vi "func-gen-simple-motor-sim.vi"(9 "Current Position Ft":dbl, 11 "Motor-Demand":dbl) -> (1 "Updated Position Ft":dbl, 3 "Velocity Ft/Sec":dbl)   [LabVIEW 2019]
uses:
  <vilib>/Rock Robotics/WPI/ThirdParty/JAS_Junk/TrajLib/VI/Util_GetTime_U32.vi
  <vilib>/Rock Robotics/WPI/ThirdParty/JAS_Junk/TrajLib/VI/TimeInterpDouble_New.vi
  <vilib>/Rock Robotics/WPI/ThirdParty/JAS_Junk/TrajLib/VI/TimeInterpDouble_AddSample.vi
  <vilib>/Rock Robotics/WPI/ThirdParty/JAS_Junk/TrajLib/VI/TimeInterpDouble_GetSample.vi
  <vilib>/Rock Robotics/WPI/ThirdParty/JAS_Junk/TrajLib/VI/TimeInterpDouble_SetMaxTime.vi
  <vilib>/Rock Robotics/WPI/ThirdParty/JAS_Junk/TrajLib/VI/TimeInterpDouble_CleanUp.vi
  <vilib>/Rock Robotics/WPI/ThirdParty/JAS_Junk/TrajLib/MathUtil_Interpolate.vi
  <vilib>/Rock Robotics/WPI/ThirdParty/JAS_Junk/TrajLib/VI/Util_GetTime_U64.vi
  <vilib>/gmath/interp.llb/Search Ordered Table.vi
  <vilib>/Rock Robotics/WPI/ThirdParty/JAS_Junk/TrajLib/Trajectory_Library.lvlib
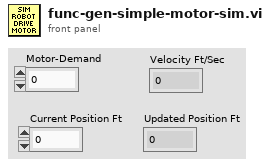
[diagram p1: front panel]
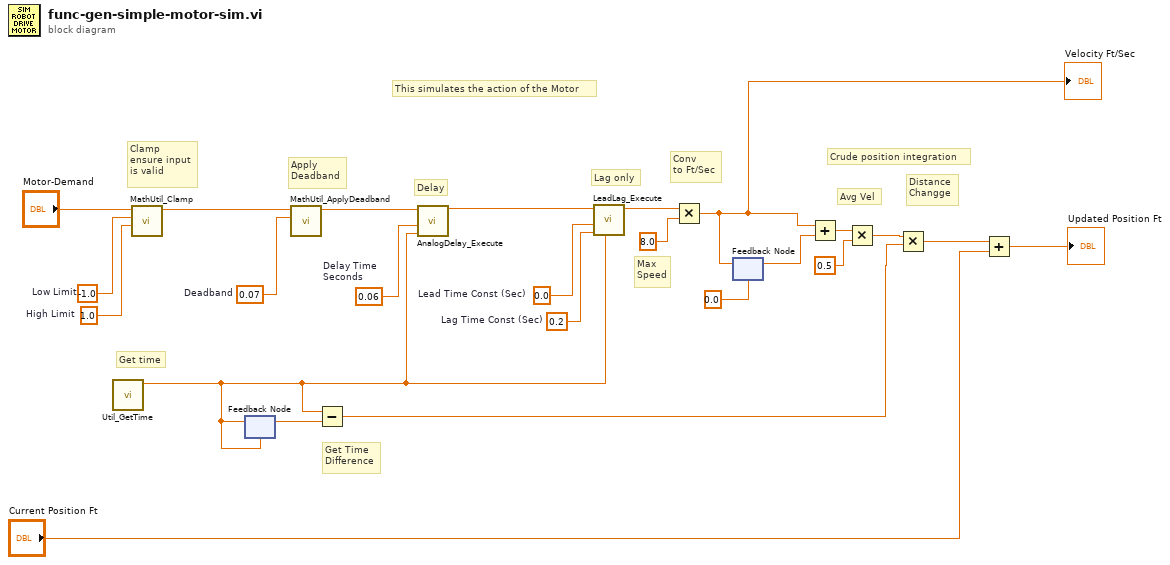
[diagram p0: block diagram]
diagram:
  w19 = 1.0  # High Limit
  w18 = -1.0  # Low Limit
  w21 = 0.2  # Lag Time Const (Sec)
  w20 = 0.0  # Lead Time Const (Sec)
  w22 = 0.06  # Delay Time Seconds
  w23 = 0.07  # Deadband
  # "Max\nSpeed"
  # "Distance\nChangge"
  # "Avg Vel"
  # "Get Time\nDifference"
  # "Get time"
  # "Conv\nto Ft/Sec"
  # "Lag only"
  # "Clamp\nensure input\nis valid"
  # "Delay"
  # "Apply\nDeadband"
  # "Crude position integration"
  # "This simulates the action of the Motor"
  n1 = call <vilib>:"Util_GetTime.vi"() -> ("FPGA_Time_Seconds"=w11:dbl)  [unwired: 9 in, 2 out]
  n2 = call <vilib>:"MathUtil_Clamp.vi"("High Limit"=w19, "Low Limit"=w18, "Value"="Motor-Demand") -> ("Result"=w13:dbl)  [unwired: 8 in]
  n3 = feedback-in #1(w11) -> ()
  n4 = feedback #1(w11) -> (w10:dbl)
  n5 = call <vilib>:"MathUtil_ApplyDeadband.vi"("Deadband"=w23, "Value"=w13) -> ("Result"=w17:dbl)  [unwired: 9 in]
  n6 = Subtract(x=w11, y=w10) -> (x-y=w3:dbl)
  n7 = call <vilib>:"AnalogDelay_Execute.vi"("Time"=w11, "Delay Time"=w22, "Input"=w17) -> ("Output"=w16:dbl)  [unwired: 7 in, 1 out]
  n8 = call <vilib>:"LeadLag_Execute.vi"("Time (Secs)"=w11, "Lag Time Const (Sec)"=w21, "Lead Time Const (Sec)"=w20, "Input"=w16) -> ("Output"=w15:dbl)  [unwired: 7 in]
  n9 = Multiply(x=w15, y=8.0) -> (x*y=w8:dbl)
  "Velocity Ft/Sec" <- w8
  n10 = feedback-in #2(w8) -> ()
  n11 = feedback #2(0.0) -> (w7:dbl)
  n12 = Add(x=w8, y=w7) -> (x+y=w6:dbl)
  n13 = Multiply(x=w6, y=0.5) -> (x*y=w4:dbl)
  n14 = Multiply(x=w4, y=w3) -> (x*y=w2:dbl)
  n15 = Add(x=w2, y="Current Position Ft") -> (x+y=→"Updated Position Ft":dbl)
